vi "Q5.vi"() -> ()   [LabVIEW 2014]
panel:
  out "reach":bool
  out "correct":bool
  in  "stop":bool
  in  "Cluster":T1
  out "total price":dbl
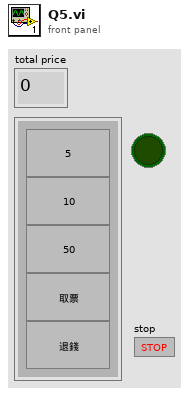
[diagram p1: front panel]
types:
  T1 = cluster{"5":bool, "10":bool, "50":bool, "conti":bool, "return":bool}
  T2 = enum16{"default", "5", "10", "50", "continue", "return"}
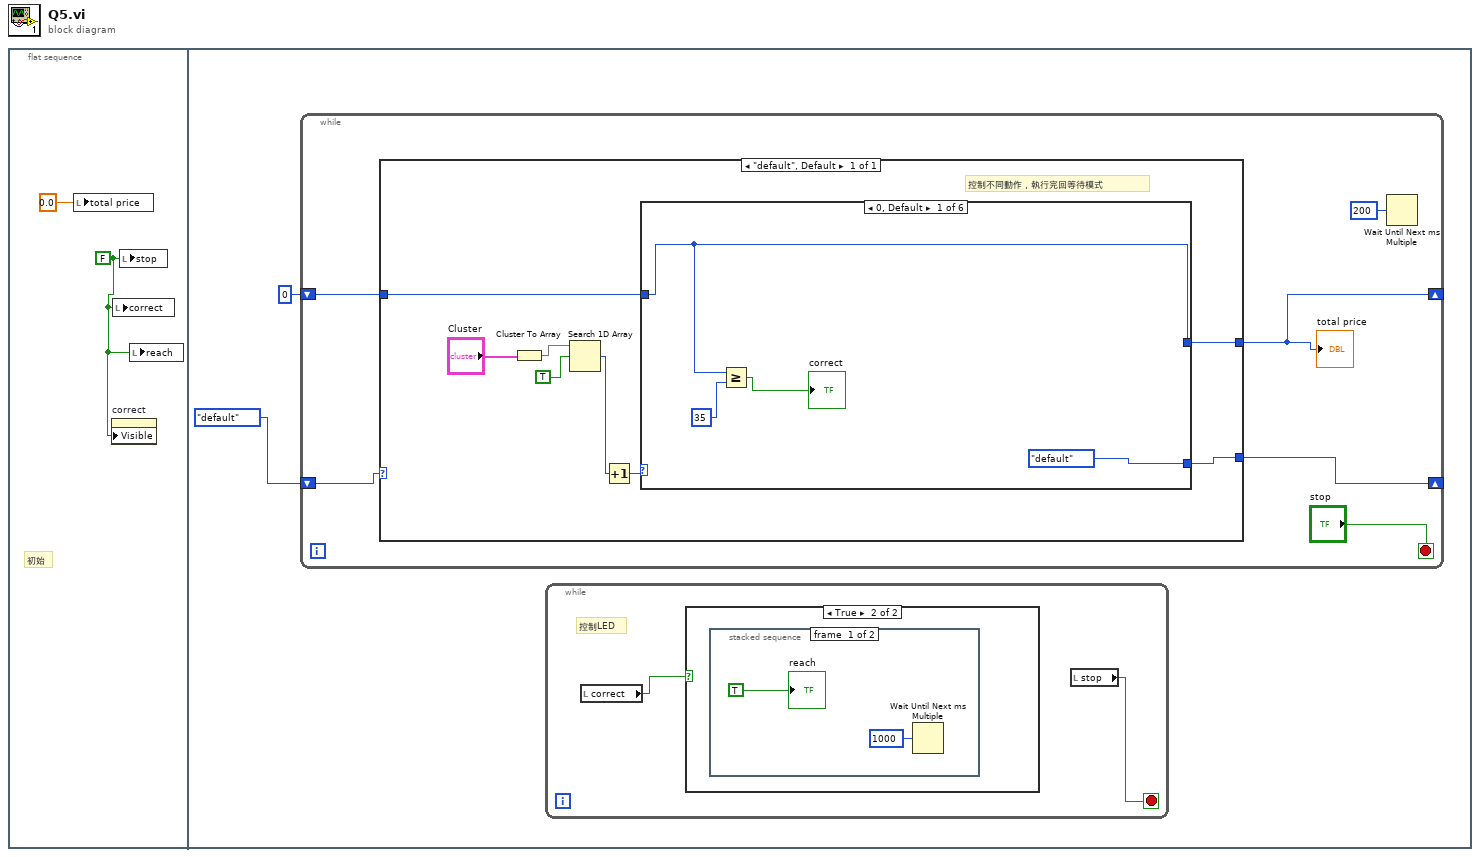
[diagram p0: block diagram]
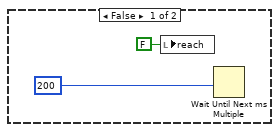
[diagram p2: hidden frame]
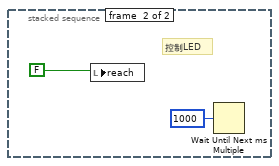
[diagram p3: hidden frame]
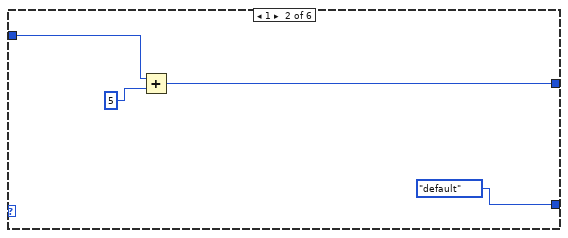
[diagram p4: hidden frame]
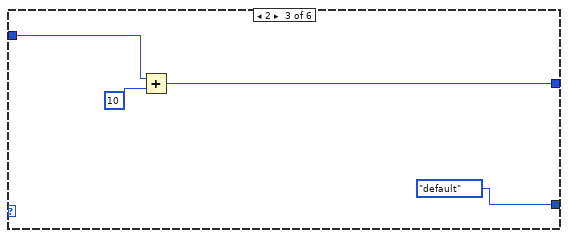
[diagram p5: hidden frame]
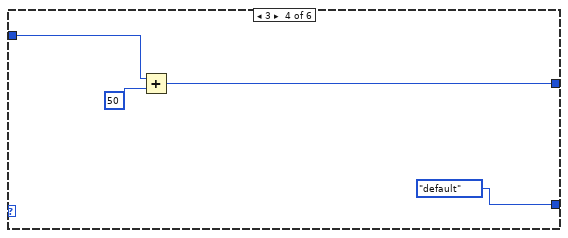
[diagram p6: hidden frame]
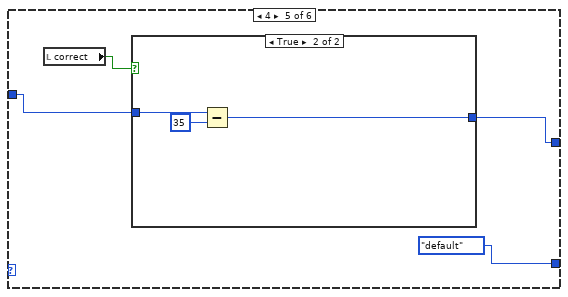
[diagram p7: hidden frame]
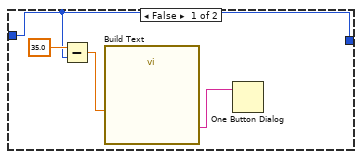
[diagram p8: hidden frame]
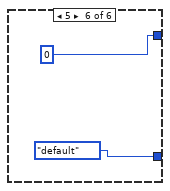
[diagram p9: hidden frame]
diagram:
  n1 = flat-sequence {
    frame #0 {
      w1 = FALSE ("stop")
      # "初始"
      n2 = local write "total price"(0.0 ("total number")) -> ()
      n3 = property on="correct" class="Bool (strict)"("Visible"=w1) -> ()  [unwired: 2 in, 2 out]
      n4 = local write "correct"(w1) -> ()
      n5 = local write "stop"(w1) -> ()
      n6 = local write "reach"(w1) -> ()
    }
    frame #1 {
      n7 = while {
        shift-right: [w17] -> _
        shift-left: T2."default" -> [w18]
        shift-right: [w16] -> _
        shift-left: 0 -> [w15]
        stop <- "stop" stop-if-true
        n8 = case shown="\"default\", Default" w18 {
          tunnel: [w25] -> w17
          tunnel: [w24] -> w16
          tunnel: w15 -> [w23]
          frame "default", Default {
            # "控制不同動作，執行完回等待模式"
            n9 = Cluster To Array(cluster="Cluster") -> (array=w22:bool[])
            n10 = Search 1D Array(1D array=w22, element=TRUE) -> (index of element=w20:i32)  [unwired: 1 in]
            n11 = Increment(x=w20) -> (x+1=w19:i32)
            n12 = case shown="0, Default" w19 {
              tunnel: [T2."default" T2."default" T2."default" T2."default" T2."default" T2."default"] -> w25
              tunnel: [w29 w33 w37 w41 w44 0] -> w24
              tunnel: w23 -> [w29 w32 w36 w40 w45 _]
              frame 0, Default {
                n13 = Greater Or Equal?(x=w29, y=35) -> (x >= y?=→"correct":bool)
              }
              frame 1 {
                n14 = Add(x=w32, y=5) -> (x+y=w33:i32)
              }
              frame 2 {
                n15 = Add(x=w36, y=10) -> (x+y=w37:i32)
              }
              frame 3 {
                n16 = Add(x=w40, y=50) -> (x+y=w41:i32)
              }
              frame 4 {
                n17 = local read "correct"() -> (w43:bool)
                n18 = case shown="True" w43 {
                  tunnel: w45 -> [w49 w53]
                  tunnel: [w49 w51] -> w44
                  frame False {
                    n19 = Subtract(x=35.0, y=w49) -> (x-y=w48:dbl)
                    n20 = call "Build Text"("money"=w48) -> ("Result"=w47:string)  [unwired: 13 in, 1 out]
                    n21 = One Button Dialog(message=w47) -> ()  [unwired: 1 in, 1 out]
                  }
                  frame True {
                    n22 = Subtract(x=w53, y=35) -> (x-y=w51:i32)
                  }
                }
              }
              frame 5 {
              }
            }
          }
        }
        "total price" <- w16
        n23 = Wait Until Next ms Multiple(millisecond multiple=u32 200) -> ()  [unwired: 1 out]
      }
      n24 = while {
        stop <- w5 stop-if-true
        # "控制LED"
        n25 = local read "correct"() -> (w6:bool)
        n26 = case shown="True" w6 {
          frame False {
            n27 = local write "reach"(FALSE ("reach")) -> ()
            n28 = Wait Until Next ms Multiple(millisecond multiple=u32 200) -> ()  [unwired: 1 out]
          }
          frame True {
            n29 = stacked-sequence {
              frame #0 {
                n30 = Wait Until Next ms Multiple(millisecond multiple=u32 1000) -> ()  [unwired: 1 out]
                "reach" <- TRUE
              }
              frame #1 {
                # "控制LED"
                n31 = local write "reach"(FALSE) -> ()
                n32 = Wait Until Next ms Multiple(millisecond multiple=u32 1000) -> ()  [unwired: 1 out]
              }
            }
          }
        }
        n33 = local read "stop"() -> (w5:bool)
      }
    }
  }
